vi "getReportImages.vi"(8 "error in (no error)":errorcluster, 9 "Diff Image":T1, 10 "Golden Image":T1, 11 "Current Image":T1) -> (0 "error out":errorcluster, 1 "Report String":string)   [LabVIEW 2018, in "Image_Diff.lvlib"]
uses:
  Image_Diff.lvlib
  <vilib>/picture/picture.llb/imagedata.ctl
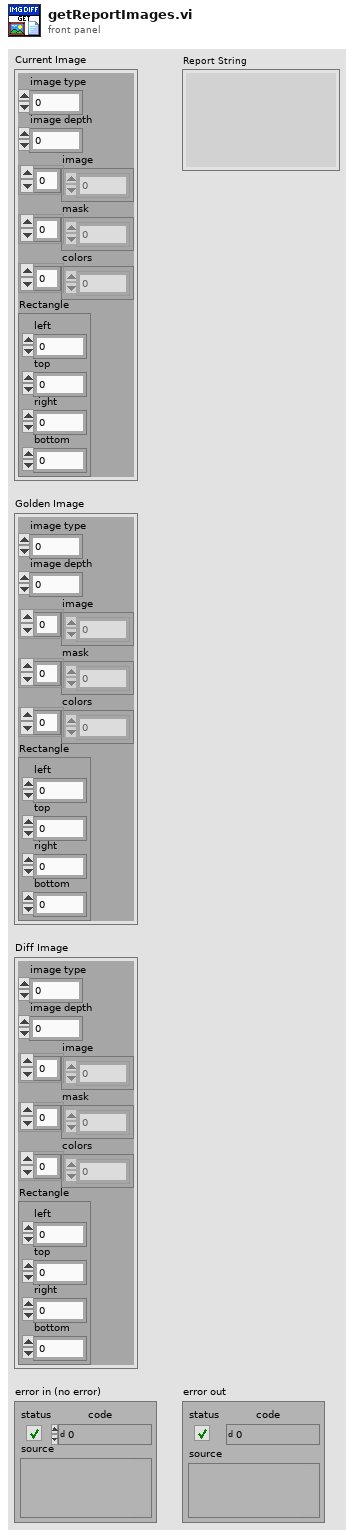
[diagram p1: front panel]
types:
  T1 = typedef "imagedata.ctl" = cluster{"image type":i32, "image depth":i32, "image":u8[], "mask":u8[], "colors":u32[], "Rectangle":cluster{"left":i16, "top":i16, "right":i16, "bottom":i16}}
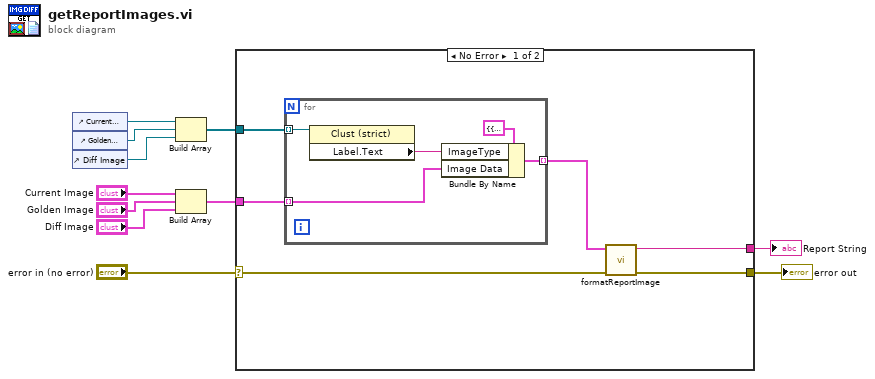
[diagram p0: block diagram]
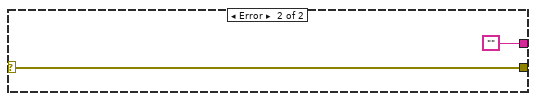
[diagram p2: hidden frame]
diagram:
  n1 = control-ref of="Current Image"() -> (w11:refnum<vi>)
  n2 = control-ref of="Golden Image"() -> (w10:refnum<vi>)
  n3 = control-ref of="Diff Image"() -> (w9:refnum<vi>)
  n4 = Build Array(w11, w10, w9) -> (w8:refnum<vi>[])
  n5 = Build Array("Current Image", "Golden Image", "Diff Image") -> (w4:T1[])
  n6 = case shown="No Error" "error in (no error)" {
    selector: "error in (no error)" -> [w13 w24]
    tunnel: w8 -> [w17 _]
    tunnel: w4 -> [w16 _]
    tunnel: [w14 ""] -> w3
    tunnel: [w12 w24] -> w1
    frame No Error {
      n7 = for {
        tunnel: w17 -> [w22] mode=indexing
        tunnel: w16 -> [w18] mode=indexing
        tunnel: [w19] -> w15 mode=indexing
        n8 = property class="Clust (strict)"(reference=w22) -> ("Label.Text"=w21:string)  [unwired: 1 in, 2 out]
        n9 = Bundle By Name(cluster=cluster{"Image Data":T1, "ImageType":string} {"Image Data"={"image type"=0, "image depth"=0, "image"=[], "mask"=[], "colors"=[], "Rectangle"={"left"=0, "top"=0, "right"=0, "bottom"=0}}, "ImageType"=""} ("Cluster"), "ImageType"=w21, "Image Data"=w18) -> (w19:cluster{"Image Data":T1, "ImageType":string})
      }
      n10 = call "formatReportImage.vi"("error in (no error)"=w13, "Image Array"=w15) -> ("error out"=w12:errorcluster, "Report String"=w14:string)  [unwired: 8 in]
    }
    frame Error {
    }
  }
  "error out" <- w1
  "Report String" <- w3
